vi "Com7 test.vi"() -> ()   [LabVIEW 2019]
uses:
  0cd483b6-e0b8-416a-96ab-2c8a4a7c8219.vi
  <vilib>/Instr/_visa.llb/VISA Configure Serial Port (Instr).vi
panel:
  in  "Send":bool
  in  "stop":bool
  out "Count Y":u32
  out "Count X":u32
  out "Y":u32
  out "X":u32
  in  "write buffer":string="M114\n"
  out "return count 2":u32
  out "Serial Settings:Number of Bytes at Serial Port":u32
  out "return count":u32
  out "read buffer":string
  out "error out":errorcluster
  # "M114"
  # "G0 X10 Y20"
  # "G0 X0 Y0"
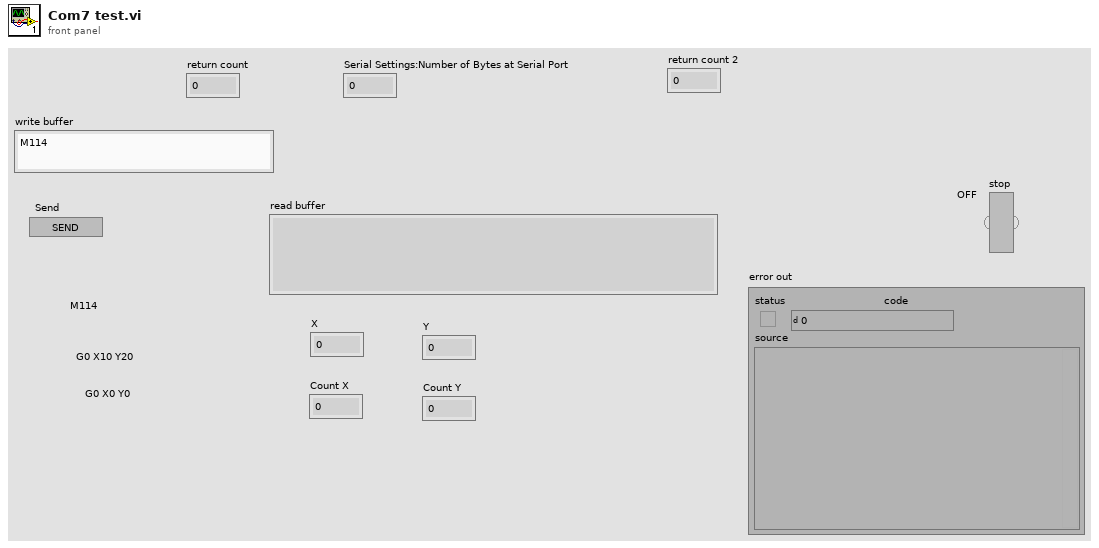
[diagram p1: front panel]
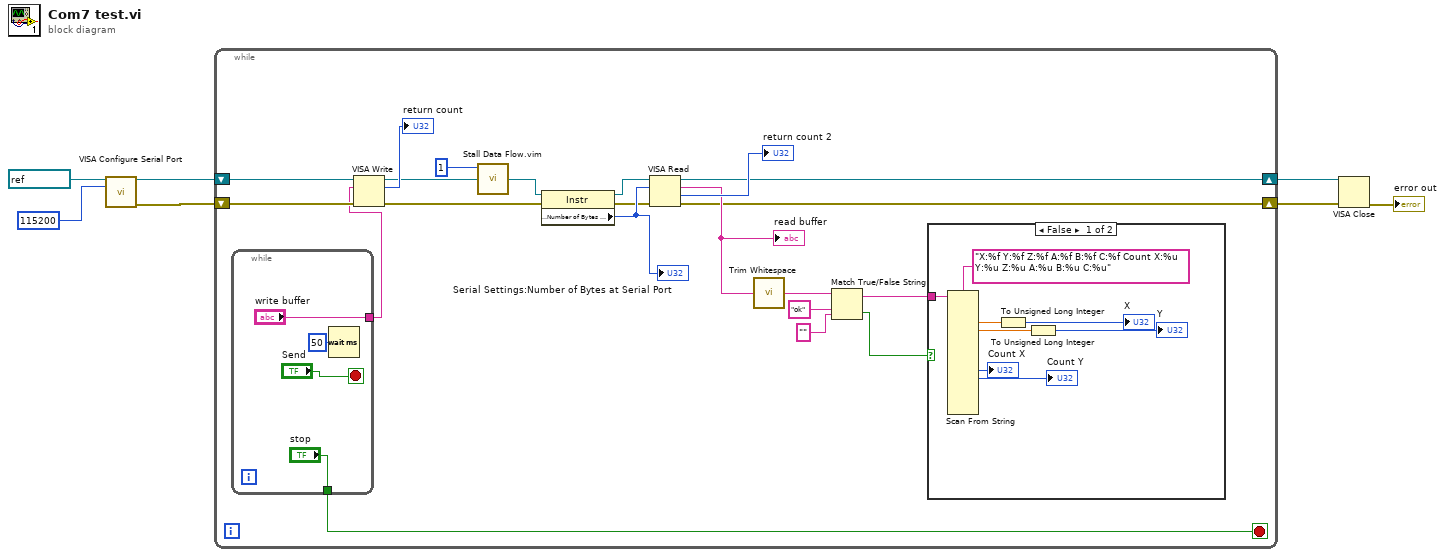
[diagram p0: block diagram]
diagram:
  n1 = call-poly "VISA Configure Serial Port"("VISA resource name"=refnum<visa-resource-name> "COM7", "baud rate (9600)"=u32 115200) -> ("VISA resource name out"=w4:refnum<visa-resource-name>, "error out"=w3:errorcluster)  [unwired: 12 in]
  n2 = while {
    shift-right: [w10] -> w2
    shift-left: w4 -> [w24]
    shift-right: [w9] -> w1
    shift-left: w3 -> [w23]
    stop <- w8 stop-if-true
    n3 = while {
      tunnel: ["write buffer"] -> w11
      tunnel: ["stop"] -> w8
      stop <- "Send" stop-if-true
      n4 = Wait (ms)(milliseconds to wait=u32 50) -> ()  [unwired: 1 out]
    }
    n5 = VISA Write(VISA resource name=w24, write buffer=w11, error in (no error)=w23) -> (VISA resource name out=w20:refnum<visa-resource-name>, return count=→"return count":u32, error out=w25:errorcluster)
    n6 = call "Stall Data Flow.vim"("value in"=w20, "milliseconds to wait"=u32 1) -> ("value out"=w19:refnum<visa-resource-name>)  [unwired: 1 out]
    n7 = property class="Instr"(reference=w19, error in=w25) -> (reference out=w28:refnum<visa-resource-name>, error out=w26:errorcluster, "Serial Settings:Number of Bytes at Serial Port"=w27:u32)
    "Serial Settings:Number of Bytes at Serial Port" <- w27
    n8 = VISA Read(VISA resource name=w28, byte count=w27, error in (no error)=w26) -> (VISA resource name out=w10:refnum<visa-resource-name>, read buffer=w17:string, return count=→"return count 2":u32, error out=w9:errorcluster)
    "read buffer" <- w17
    n9 = call <vilib>:"Trim Whitespace.vi"("string"=w17) -> ("trimmed string"=w16:string)  [unwired: 1 in]
    n10 = Match True/False String(2:"" ("false string"), 3:"ok" ("true string"), 4:w16) -> (0:w14:bool, 1:w13:string)
    n11 = case shown="False" w14 {
      tunnel: w13 -> [w33 _]
      frame False {
        n12 = Scan From String(format string="X:%f Y:%f Z:%f A:%f B:%f C:%f Count X:%u Y:%u Z:%u A:%u B:%u C:%u", input string=w33) -> (output 1=w37:dbl, output 2=w35:dbl, output 7=→"Count X":u32, output 8=→"Count Y":u32)  [unwired: 22 in, 3 out]
        n13 = To Unsigned Long Integer(number=w37) -> (unsigned 32bit integer=→"X":u32)
        n14 = To Unsigned Long Integer(number=w35) -> (unsigned 32bit integer=→"Y":u32)
      }
      frame True {
      }
    }
  }
  n15 = VISA Close(VISA resource name=w2, error in (no error)=w1) -> (error out=→"error out":errorcluster)
